vi "Day 2.vi"() -> ()   [LabVIEW 2019]
panel:
  in  "Error In":errorcluster
  in  "Relative Path to Raw Data":string
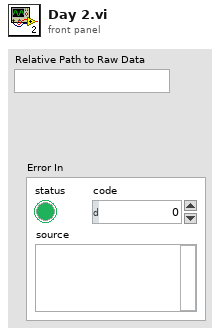
[diagram p1: front panel]
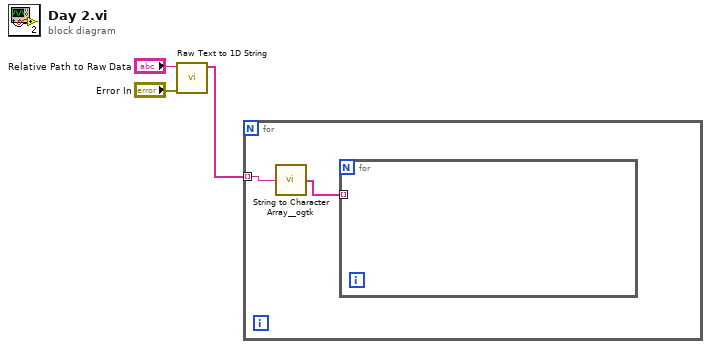
[diagram p0: block diagram]
diagram:
  n1 = call "Raw Text to 1D String.vi"("Error In"="Error In", "Relative Path to Input File"="Relative Path to Raw Data") -> ("1D String Array"=w1:string[])  [unwired: 8 in, 1 out]
  n2 = for {
    tunnel: w1 -> [w5] mode=indexing
    n3 = call <userlib>:"String to Character Array__ogtk.vi"("Input String"=w5) -> ("Character Array"=w4:string[])
    n4 = for {
      tunnel: w4 -> [_] mode=indexing
    }
  }
